vi "DSF.Memory.Cache.Transfer.Set Channel Configuration.vi"(8 "error in (no error)":errorcluster, 10 "Channel Configuration":T1[](array[typedef]) {"count" format="%d elements"; "offset" format="%d bytes"}, 11 "Transfer Cache in":refnum<class "DSF.Memory.Cache.Transfer.lvclass">) -> (0 "error out":errorcluster, 3 "Transfer Cache out":refnum<class "DSF.Memory.Cache.Transfer.lvclass">)   [LabVIEW 2016, in "DSF.Memory.lvlib" / "DSF.Memory.Cache.Transfer.lvclass"]
uses:
  DSF.Memory.Cache.Transfer.lvclass
  Typedefs/DSF.Common.DataType.ctl
  DSF.Common.lvlib
  Typedefs/DSF.Memory.Buffer Channel Configuration.ctl
  DSF.Memory.lvlib
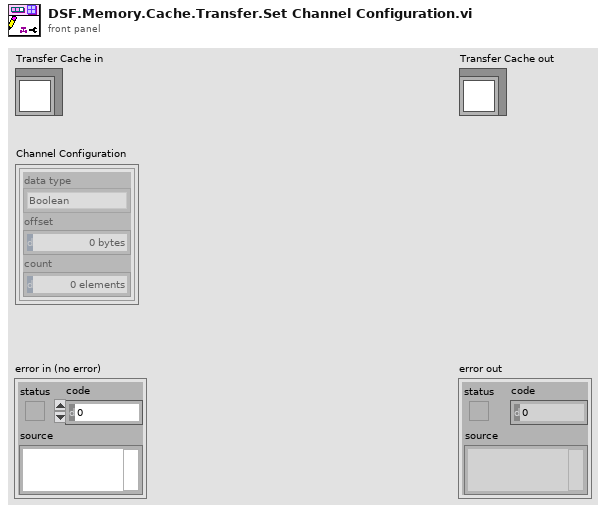
[diagram p1: front panel]
types:
  T1 = typedef "DSF.Memory.lvlib/DSF.Memory.Buffer Channel Configuration.ctl" = cluster{"data type":T2, "offset":u64, "count":u64}
  T2 = typedef "DSF.Common.lvlib/DSF.Common.DataType.ctl" = enum8{"Boolean", "Single", "Double", "Int8", "Int16", "Int32", "Int64", "UInt8", "UInt16", "UInt32", "UInt64"}
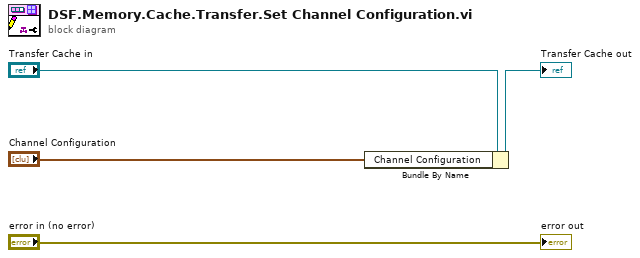
[diagram p0: block diagram]
diagram:
  n1 = Bundle By Name(cluster="Transfer Cache in", "Channel Configuration"="Channel Configuration") -> (→"Transfer Cache out":refnum<class "DSF.Memory.Cache.Transfer.lvclass">)
  "error out" <- "error in (no error)"
